vi "Read from Stream.vi"(10 "Stream in":refnum<class "Stream.lvclass">, 11 "LabVIEW JSON in":refnum<class "LabVIEW JSON.lvclass">) -> (0 "error out":errorcluster, 2 "Message Data":T1)   [LabVIEW 2020, in "Stream-Simple-Msg.lvlib" / "LabVIEW JSON.lvclass"]
uses:
  LabVIEW JSON.lvclass
  <vilib>/IlluminatedG/lv-stream/stream/Stream.lvclass
  Message/Message Data.ctl
  Message/Message___.lvclass
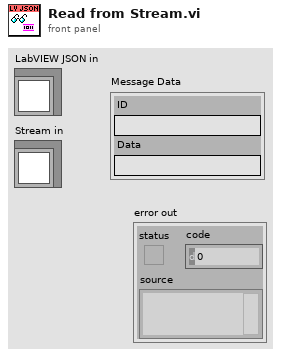
[diagram p1: front panel]
types:
  T1 = typedef "Stream-Simple-Msg.lvlib/Message___.lvclass/Message Data.ctl" = cluster{"ID":string, "Data":string}
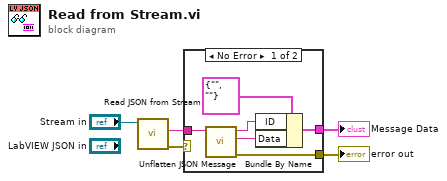
[diagram p0: block diagram]
diagram:
  n1 = call "Read JSON from Stream.vi"("Stream in"="Stream in") -> ("error out"=w3:errorcluster, "Data"=w4:string)  [unwired: 9 in]
  n2 = case shown="No Error" w3 {
    selector: w3 -> [_ w12]
    tunnel: w4 -> [w11 _]
    tunnel: [w10 w12] -> w2
    tunnel: [w8 _] -> w1
    frame No Error {
      n3 = call "Unflatten JSON Message.vi"("Raw Data"=w11) -> ("error out"=w10:errorcluster, "JSON Value"=w6:string, "ID"=w7:string)  [unwired: 7 in, 1 out]
      n4 = Bundle By Name(cluster=T1 {"ID"="", "Data"=""} ("Message Data"), "ID"=w7, "Data"=w6) -> (w8:T1)
    }
    frame Error {
    }
  }
  "error out" <- w2
  "Message Data" <- w1
